vi "ReportPart_A170316-11.vi"(6 "试验项目":enum32{"磨合", "空载检测", "啮合间隙"}(ring), 8 "error in":errorcluster, 9 "索引":i32, 10 "合格":T1, 11 "report in":refnum<class "NI_report.lvclass">) -> (0 "error out":errorcluster, 3 "report out":refnum<class "NI_report.lvclass">)   [LabVIEW 2020]
uses:
  <vilib>/Utility/NIReport.llb/NI_report.lvclass
  OK.ctl
  <vilib>/Utility/NIReport.llb/image depth.ctl
  <vilib>/addons/_office/_exclsub.llb/font.ctl
  Global_Variable/A170316-11.vi
  <vilib>/Utility/NIReport.llb/Append Report Text (str wrap).vi
  Global_Variable/Global.vi
  <vilib>/addons/_office/word.llb/Word Easy Table (str).vi
  <vilib>/Utility/NIReport.llb/NI_ReportGenerationCore.lvlib
  <vilib>/Utility/NIReport.llb/Word/NI_Word.lvclass
  <vilib>/addons/_office/NI_ReportGenerationToolkit.lvlib
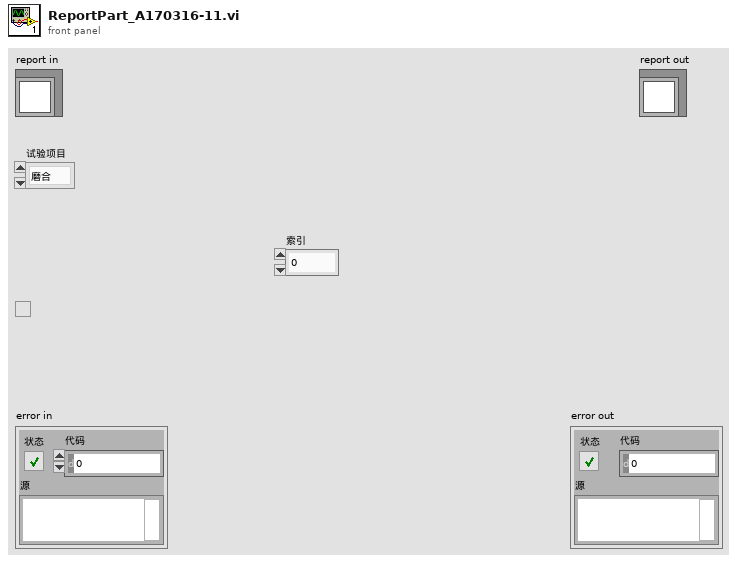
[diagram p1: front panel]
types:
  T1 = typedef "OK.ctl" = bool
  T2 = cluster{"Italic":enum16{"Italic Unchanged", "Italic On", "Italic Off"}, "Strike Through":enum16{"Strike Through Unchanged", "Strike Through On", "Strike Through Off"}, "Underline":enum16{"Underline Unchanged", "Underline On", "Underline Off"}, "Bold":enum16{"Bold Unchanged", "Bold On", "Bold Off"}}
  T3 = cluster{"Charset (-1)":i16, "Weight (-1)":i16, "Name":string, "Size":string}
  T4 = typedef "NI_ReportGenerationToolkit.lvlib/font.ctl" = cluster{"font name":string, "font size":dbl, "bold":u16, "italic":u16, "underline":u16, "strike through":u16, "font color":u32}
  T5 = typedef "NI_ReportGenerationCore.lvlib/image depth.ctl" = u16
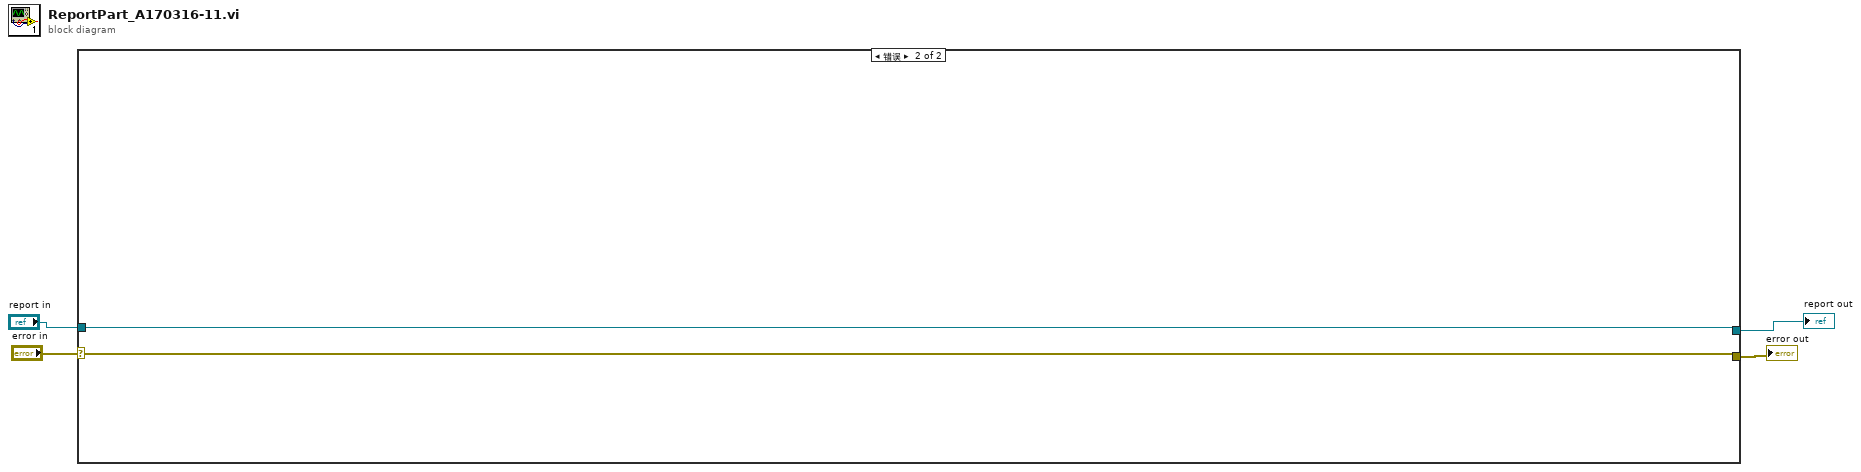
[diagram p0: block diagram]
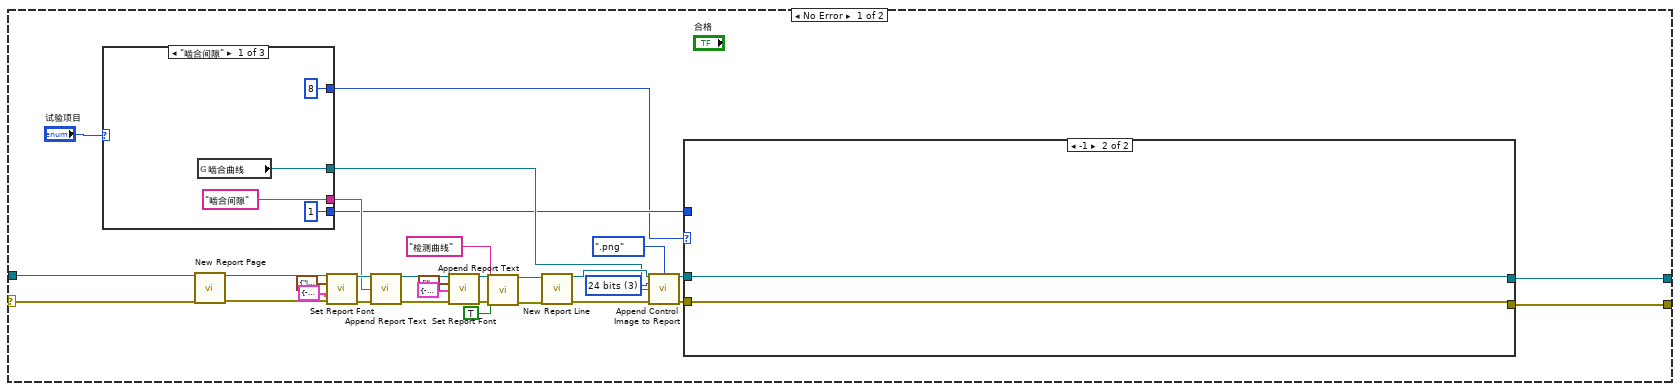
[diagram p2: hidden frame]
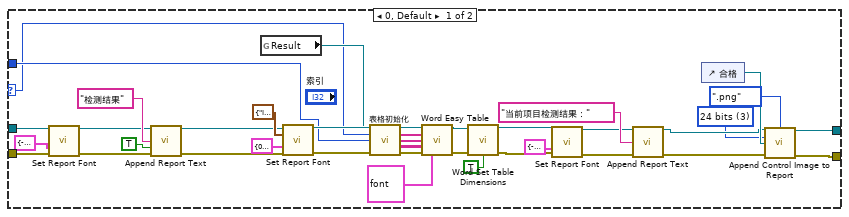
[diagram p3: hidden frame]
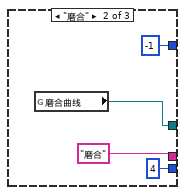
[diagram p4: hidden frame]
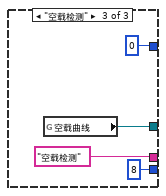
[diagram p5: hidden frame]
diagram:
  n1 = case shown="错误" "error in" {
    selector: "error in" -> [w14 w87]
    tunnel: "report in" -> [w7 w88]
    tunnel: [w6 w88] -> w2
    tunnel: [w5 w87] -> w1
    frame No Error {
      w33 = T5 3 items=["B&W", "4 bits", "8 bits", "24 bits"] ("image depth")
      n2 = case shown="\"啮合间隙\"" "试验项目" {
        tunnel: [w75 w79 w83] -> w10
        tunnel: ["啮合间隙" ("text") "磨合" ("text") "空载检测" ("text")] -> w27
        tunnel: [1 ("长度") 4 ("长度") 8 ("长度")] -> w9
        tunnel: [8 ("长度") -1 ("长度") 0 ("长度")] -> w8
        frame "啮合间隙" {
          n3 = global read "A170316-11.vi" "啮合曲线"() -> (w75:refnum<vi>)
        }
        frame "磨合" {
          n4 = global read "A170316-11.vi" "磨合曲线"() -> (w79:refnum<vi>)
        }
        frame "空载检测" {
          n5 = global read "A170316-11.vi" "空载曲线"() -> (w83:refnum<vi>)
        }
      }
      n6 = call-dynamic "New Report Page.vi"("report in"=w7, "error in (no error)"=w14) -> ("report out"=w12:refnum<class "NI_report.lvclass">, "error out"=w13:errorcluster)  [unwired: 12 in]
      n7 = call-dynamic "Set Report Font.vi"("report in"=w12, "text options"=T2 {"Italic"=enum."Italic Unchanged", "Strike Through"=enum."Strike Through Unchanged", "Underline"=enum."Underline Unchanged", "Bold"=enum."Bold On"}, "font settings"=T3 {"Charset (-1)"=-1, "Weight (-1)"=-1, "Name"="楷体", "Size"="16 "}, "error in (no error)"=w13) -> ("report out"=w32:refnum<class "NI_report.lvclass">, "error out"=w31:errorcluster)  [unwired: 9 in, 1 out]
      n8 = call-poly <vilib>:"Append Report Text.vi"("report in"=w32, "text"=w27, "error in (no error)"=w31) -> ("report out"=w24:refnum<class "NI_report.lvclass">, "error out"=w23:errorcluster)  [unwired: 9 in, 2 out]
      n9 = call-dynamic "Set Report Font.vi"("report in"=w24, "text options"=T2 {"Italic"=enum."Italic Unchanged", "Strike Through"=enum."Strike Through Unchanged", "Underline"=enum."Underline Unchanged", "Bold"=enum."Bold Off"}, "font settings"=T3 {"Charset (-1)"=-1, "Weight (-1)"=-1, "Name"="宋体", "Size"="12 "}, "error in (no error)"=w23) -> ("report out"=w20:refnum<class "NI_report.lvclass">, "error out"=w17:errorcluster)  [unwired: 9 in, 1 out]
      n10 = call-poly <vilib>:"Append Report Text.vi"("report in"=w20, "text"="检测曲线", "append on new line? (F)"=TRUE, "error in (no error)"=w17) -> ("report out"=w19:refnum<class "NI_report.lvclass">, "error out"=w18:errorcluster)  [unwired: 8 in, 2 out]
      n11 = call-dynamic "New Report Line.vi"("report in"=w19, "error in (no error)"=w18) -> ("report out"=w34:refnum<class "NI_report.lvclass">, "error out"=w35:errorcluster)  [unwired: 12 in]
      n12 = call-dynamic "Append Control Image to Report.vi"("report in"=w34, "image file type (.jpg)"=enum16{".jpg", ".png"}.".png", "image depth"=w33, "ctrl reference"=w10, "error in (no error)"=w35) -> ("report out"=w29:refnum<class "NI_report.lvclass">, "error out"=w28:errorcluster)  [unwired: 7 in, 2 out]
      n13 = case shown="-1" w8 {
        selector: w8 -> [w49 _]
        tunnel: w29 -> [w68 w74]
        tunnel: w28 -> [w66 w73]
        tunnel: w9 -> [w50 _]
        tunnel: [w37 w74] -> w6
        tunnel: [w36 w73] -> w5
        frame 0, Default {
          w39 = T5 3 items=["B&W", "4 bits", "8 bits", "24 bits"] ("image depth")
          n14 = call-dynamic "Set Report Font.vi"("report in"=w68, "font settings"=T3 {"Charset (-1)"=-1, "Weight (-1)"=-1, "Name"="宋体", "Size"="12 "}, "error in (no error)"=w66) -> ("report out"=w69:refnum<class "NI_report.lvclass">, "error out"=w67:errorcluster)  [unwired: 10 in, 1 out]
          n15 = call-poly <vilib>:"Append Report Text.vi"("report in"=w69, "text"="检测结果", "append on new line? (F)"=TRUE, "error in (no error)"=w67) -> ("report out"=w53:refnum<class "NI_report.lvclass">, "error out"=w52:errorcluster)  [unwired: 8 in, 2 out]
          n16 = global read "Global.vi" "Result"() -> (w51:refnum<vi>)
          n17 = call-dynamic "Set Report Font.vi"("report in"=w53, "text options"=T2 {"Italic"=enum."Italic Unchanged", "Strike Through"=enum."Strike Through Unchanged", "Underline"=enum."Underline Unchanged", "Bold"=enum."Bold Unchanged"}, "font settings"=T3 {"Charset (-1)"=0, "Weight (-1)"=-1, "Name"="微软雅黑", "Size"="12 "}, "error in (no error)"=w52) -> ("report out"=w55:refnum<class "NI_report.lvclass">, "error out"=w54:errorcluster)  [unwired: 9 in, 1 out]
          n18 = call "表格初始化.vi"("表格引用"=w51, "索引"=w49, "长度"=w50, "错误输入（无错误）"=w54) -> ("行首字符串[]"=w57:string[], "列首字符串[]"=w56:string[], "文本数据"=w59:string[][], "错误输出"=w62:errorcluster)  [unwired: 7 in, 1 out]
          n19 = call-poly <vilib>:"Word Easy Table.vi"("report in"=w55, "row headers"=w57, "column headers"=w56, "data"=w59, "error in (no error)"=w62, "font"=T4 {"font name"="宋体", "font size"=12.0, "bold"=2, "italic"=2, "underline"=2, "strike through"=2, "font color"=16777216}) -> ("report out"=w60:refnum<class "NI_report.lvclass">, "error out"=w61:errorcluster)  [unwired: 7 in, 1 out]
          n20 = call <vilib>:"Word Set Table Dimensions.vi"("report in"=w60, "error in (no error)"=w61, "fit to page width? (F)"=TRUE) -> ("report out"=w47:refnum<class "NI_report.lvclass">, "error out"=w45:errorcluster)  [unwired: 11 in]
          n21 = call-dynamic "Set Report Font.vi"("report in"=w47, "font settings"=T3 {"Charset (-1)"=-1, "Weight (-1)"=-1, "Name"="宋体", "Size"="16 "}, "error in (no error)"=w45) -> ("report out"=w43:refnum<class "NI_report.lvclass">, "error out"=w44:errorcluster)  [unwired: 10 in, 1 out]
          n22 = call-poly <vilib>:"Append Report Text.vi"("report in"=w43, "text"="当前项目检测结果：", "error in (no error)"=w44) -> ("report out"=w41:refnum<class "NI_report.lvclass">, "error out"=w38:errorcluster)  [unwired: 9 in, 2 out]
          n23 = control-ref of="合格"() -> (w42:refnum<vi>)
          n24 = call-dynamic "Append Control Image to Report.vi"("report in"=w41, "image file type (.jpg)"=enum16{".jpg", ".png"}.".png", "image depth"=w39, "ctrl reference"=w42, "error in (no error)"=w38) -> ("report out"=w37:refnum<class "NI_report.lvclass">, "error out"=w36:errorcluster)  [unwired: 7 in, 2 out]
        }
        frame -1 {
        }
      }
    }
    frame Error {
    }
  }
  "error out" <- w1
  "report out" <- w2
